vi "ukol1.vi"() -> ()   [LabVIEW 2023]
uses:
  <vilib>/Analysis/4window.llb/windowTd.ctl
  <vilib>/measure/maspectr.llb/FFT Spectrum (Mag-Phase) for 1 Chan.vi
  <vilib>/measure/NI_MABase.lvlib
  <vilib>/measure/NI_MAPro.lvlib
  <vilib>/Analysis/NI_AALPro.lvlib
panel:
  out "x*y 2":dbl
  out "x/y":dbl
  in  "stop":bool
  in  "amplitude":dbl=1.0 format="%0.2p"
  in  "frequency":dbl=10.0 format="%0.2p"
  out "Waveform Graph 3":cluster{"f0":dbl, "df":dbl, "phase":dbl[]}(graph)
  out "Waveform Graph 2":cluster{"f0":dbl, "df":dbl, "magnitude":dbl[]}(graph)
  out "x*y":dbl
  out "Waveform Graph":waveform(dbl)[](graph)
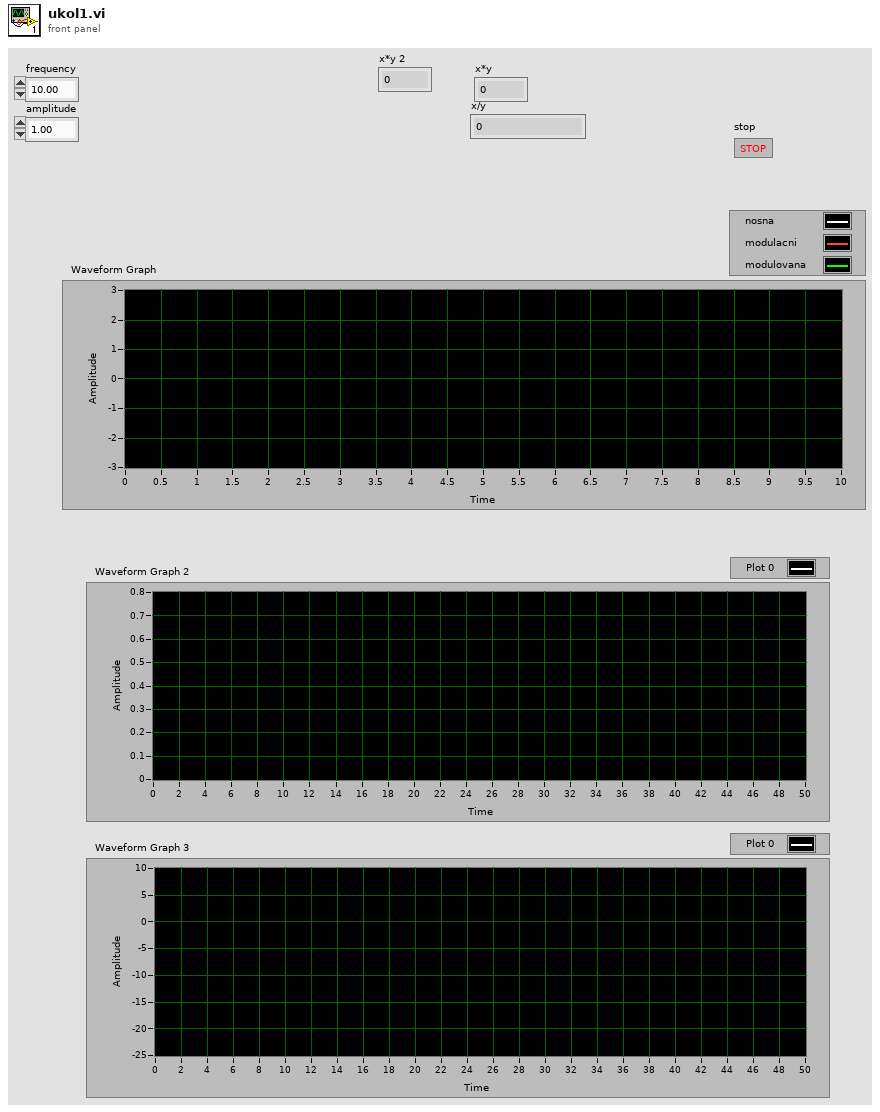
[diagram p1: front panel]
types:
  T1 = cluster{"dB On (F)":bool, "unwrap phase (F)":bool, "convert to degree (F)":bool}
  T2 = typedef "NI_AALPro.lvlib/windowTd.ctl" = u32
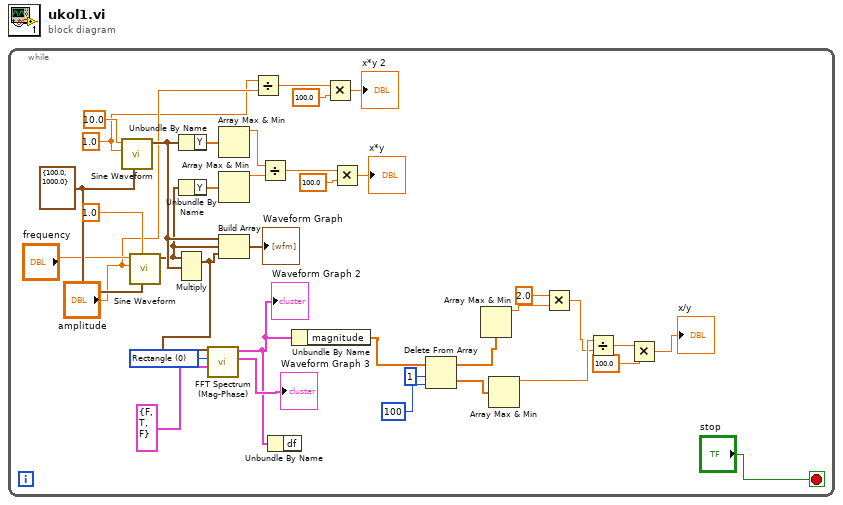
[diagram p0: block diagram]
diagram:
  n1 = while {
    stop <- "stop" stop-if-true
    w21 = T2 0 items=["Rectangle"=0, "Hanning"=1, "Hamming"=2, "Blackman-Harris"=3, "Exact Blackman"=4, "Blackman"=5, "Flat Top"=6, "4 Term B-Harris "=7, "7 Term B-Harris"=8, "Low Sidelobe"=9, "Blackman Nuttall"=11, "Triangle"=30, "Bartlett-Hanning"=31, "Bohman"=32, "Parzen"=33, "Welch"=34, "Kaiser"=60, "Dolph-Chebyshev"=61, "Gaussian"=62] ("window")
    w36 = cluster{"Fs":dbl, "#s":dbl} {"Fs"=100.0, "#s"=1000.0} ("sampling info")
    w1 = 1.0 ("amplitude")
    n2 = call <vilib>:"Sine Waveform.vi"("sampling info"=w36, "amplitude"=w1, "frequency"=10.0) -> ("signal out"=w34:waveform(dbl))  [unwired: 7 in, 1 out]
    n3 = call <vilib>:"Sine Waveform.vi"("offset"=1.0, "sampling info"=w36, "amplitude"="amplitude", "frequency"="frequency") -> ("signal out"=w26:waveform(dbl))  [unwired: 6 in, 1 out]
    n4 = Multiply(1:w34, 2:w26) -> (0:w23:waveform(dbl))  [unwired: 1 in, 1 out]
    n5 = Unbundle By Name(w34) -> ("Y"=w33:dbl[])
    n6 = Unbundle By Name(w26) -> ("Y"=w32:dbl[])
    n7 = call-poly <vilib>:"FFT Spectrum (Mag-Phase).vi"("view"=T1 {"dB On (F)"=FALSE, "unwrap phase (F)"=TRUE, "convert to degree (F)"=FALSE}, "window"=w21, "time signal"=w23) -> ("phase"=→"Waveform Graph 3":cluster{"f0":dbl, "df":dbl, "phase":dbl[]}, "magnitude"=w20:cluster{"f0":dbl, "df":dbl, "magnitude":dbl[]})  [unwired: 4 in, 3 out]
    "Waveform Graph 2" <- w20
    n8 = Array Max & Min(array=w33) -> (max value=w28:dbl)  [unwired: 3 out]
    n9 = Array Max & Min(array=w32) -> (max value=w27:dbl)  [unwired: 3 out]
    n10 = Build Array(w34, w26, w23) -> (→"Waveform Graph":waveform(dbl)[])
    n11 = Divide(x=w1, y="amplitude") -> (x/y=w6:dbl)
    n12 = Divide(x=w28, y=w27) -> (x/y=w31:dbl)
    n13 = Unbundle By Name(w20) -> ()  [unwired: 1 out]
    n14 = Unbundle By Name(w20) -> ("magnitude"=w18:dbl[])
    n15 = Multiply(x=w6, y=100.0) -> (x*y=→"x*y 2":dbl)
    n16 = Multiply(x=w31, y=100.0) -> (x*y=→"x*y":dbl)
    n17 = Delete From Array(array=w18, length=1, index=100 ("length")) -> (deleted portion=w15:dbl[], array with subset deleted=w17:dbl[])
    n18 = Array Max & Min(array=w17) -> (max value=w13:dbl)  [unwired: 3 out]
    n19 = Array Max & Min(array=w15) -> (max value=w11:dbl)  [unwired: 3 out]
    n20 = Multiply(x=2.0, y=w13) -> (x*y=w10:dbl)
    n21 = Divide(x=w11, y=w10) -> (x/y=w9:dbl)
    n22 = Multiply(x=w9, y=100.0) -> (x*y=→"x/y":dbl)
  }
